vi "Longer Pump dLSP501 Read System Information.vi"(0 "VISA resource name":refnum<visa-resource-name>="COM1" caption="VISA资源名", 7 "Comm. Config.":T1={"Address"=1, "Baud Rate"=115200, "Parity"=0} caption="通讯设置" {"Parity" items=["无校验", "奇校验", "偶校验", "标记", "空格"]; "Baud Rate" items=["1200"=1200, "2400"=2400, "9600"=9600, "19200"=19200, "38400"=38400, "57600"=57600, "115200"=115200]}) -> (6 "Model Number":string caption="设备型号", 8 "Serial Number":string caption="序 列 号", 10 "Firmware Revision":string caption="固件版本")   [LabVIEW 2023, in "Longer Pump dLSP501 Series.lvlib"]
uses:
  <instrlib>/Longer Pump dLSP501 Modbus RTU Series/Longer Pump dLSP501 Series.lvlib
  <vilib>/NI/Modbus Library/API/Master/Modbus Master.lvclass
  C:/Program Files/National Instruments/LabVIEW 2023/vi.lib/NI/Modbus Library/API/Modbus API.lvclass
  <instrlib>/Longer Pump dLSP501 Modbus RTU Series/Private/Initialize - Integrated Address.vi
  <vilib>/NI/Modbus Library/API/Modbus API.lvclass
panel:
  out "Error out":errorcluster caption="错误输出"
  in  "Error in":errorcluster caption="错误输入"
  in  "Open Port":bool caption="打开串口"
  out "Hardware Revision":string caption="硬件版本"
  in  "Close Port":bool caption="关闭串口"
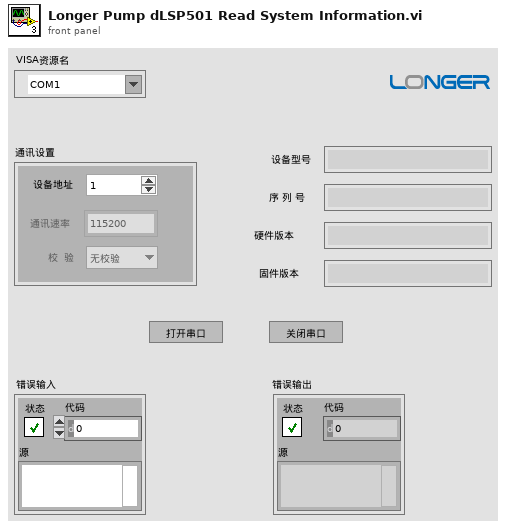
[diagram p1: front panel]
types:
  T1 = cluster{"Address":u8, "Baud Rate":u32, "Parity":u16}
  T2 = enum8{"Enabled", "Disabled", "Disabled and Grayed Out"}
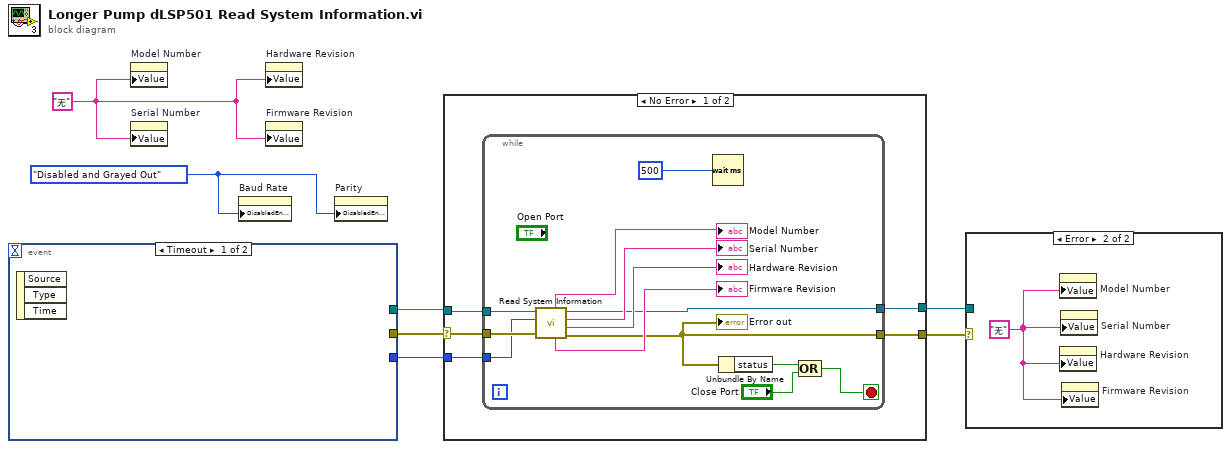
[diagram p0: block diagram]
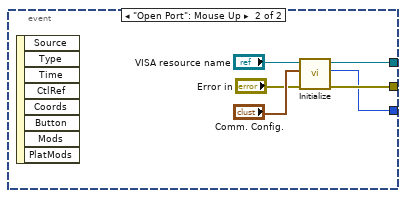
[diagram p2: hidden frame]
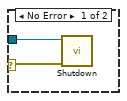
[diagram p4: hidden frame]
diagram:
  w1 = "无"
  w2 = T2."Disabled and Grayed Out" ("禁用")
  n1 = event shown="[0] Timeout" {
    selector: _ -> [_ _]
    dyn-events: _ -> [_ _]
    timeout: _ -> [_ _]
    tunnel: [_ w11] -> w5
    tunnel: [_ w10] -> w4
    tunnel: [_ w9] -> w3
    event Timeout {
      n2 = event-data() -> ()  [unwired: 1 in, 3 out]
    }
    event "Open Port": Mouse Up {
      n3 = event-data() -> ()  [unwired: 1 in, 8 out]
      n4 = call-poly <instrlib>:"Initialize.vi"("Error in"="Error in", "Comm. Config"="Comm. Config.", "VISA resource name"="VISA resource name") -> ("Error out"=w11:errorcluster, "Channel"=w10:i32, "serial master instance"=w9:refnum<class "Modbus Master.lvclass">)  [unwired: 5 in]
    }
  }
  n5 = property on="Model Number" class="Str"("Value"=w1) -> ()  [unwired: 2 in, 2 out]
  n6 = property on="Serial Number" class="Str"("Value"=w1) -> ()  [unwired: 2 in, 2 out]
  n7 = property on="Baud Rate" class="Ring (strict)"("DisabledEnum"=w2) -> ()  [unwired: 2 in, 2 out]
  n8 = property on="Hardware Revision" class="Str"("Value"=w1) -> ()  [unwired: 2 in, 2 out]
  n9 = property on="Firmware Revision" class="Str"("Value"=w1) -> ()  [unwired: 2 in, 2 out]
  n10 = property on="Parity" class="Ring (strict)"("DisabledEnum"=w2) -> ()  [unwired: 2 in, 2 out]
  n11 = case shown="No Error" w5 {
    selector: w5 -> [w15 w32]
    tunnel: w3 -> [w18 w33]
    tunnel: [w17 w33] -> w7
    tunnel: [w16 w32] -> w6
    tunnel: w4 -> [w14 _]
    frame No Error {
      n12 = while {
        tunnel: w18 -> [w31]
        tunnel: [w25] -> w17
        tunnel: [w19] -> w16
        tunnel: w15 -> [w21]
        tunnel: w14 -> [w20]
        stop <- w22 stop-if-true
        n13 = call <instrlib>:"Read System Information.vi"("Error in"=w21, "Channel"=w20, "Modbus master in"=w31) -> ("Error out"=w19:errorcluster, "Hardware Revision"=→"Hardware Revision":string, "Serial Number"=→"Serial Number":string, "Modbus instance out"=w25:refnum<class "Modbus API.lvclass">, "Firmware Revision"=→"Firmware Revision":string, "Model Number"=→"Model Number":string)  [unwired: 3 in]
        "Error out" <- w19
        n14 = Wait (ms)(milliseconds to wait=u32 500 ("等待时间（毫秒）")) -> ()  [unwired: 1 out]
        n15 = Unbundle By Name(w19) -> ("status"=w24:bool)
        n16 = Compound Arithmetic op=OR ("复合运算")(w24, "Close Port") -> (w22:bool)
      }
    }
    frame Error {
    }
  }
  n17 = case shown="Error" w6 {
    selector: w6 -> [w34 _]
    tunnel: w7 -> [w35 _]
    frame No Error {
      n18 = call-dynamic "Shutdown.vi"("error in"=w34, "Modbus instance in"=w35) -> ()  [unwired: 9 in, 1 out]
    }
    frame Error {
      w36 = "无"
      n19 = property on="Model Number" class="Str"("Value"=w36) -> ()  [unwired: 2 in, 2 out]
      n20 = property on="Hardware Revision" class="Str"("Value"=w36) -> ()  [unwired: 2 in, 2 out]
      n21 = property on="Serial Number" class="Str"("Value"=w36) -> ()  [unwired: 2 in, 2 out]
      n22 = property on="Firmware Revision" class="Str"("Value"=w36) -> ()  [unwired: 2 in, 2 out]
    }
  }
